vi "Anritsu VNA Set Frequency On-Off.vi"(7 "Anritsu VNA":T1, 8 "error in (no error)":errorcluster, 10 "Blank Frequencies (F)":bool, 11 "VISA Resource Name":refnum<visa-resource-name>) -> (0 "error out":errorcluster, 3 "dup VISA Resource Name":refnum<visa-resource-name>)   [LabVIEW 2011]
doc: "This VI for the HP8753B Network Analyzers reads the stimulus values. Except when performing log sweeps and freq list sweeps, this VI uses the start and stop values and the number of points to calcuate the stimulus values."
uses:
  TypeDefs/Anritsu VNA Instrument Info.ctl
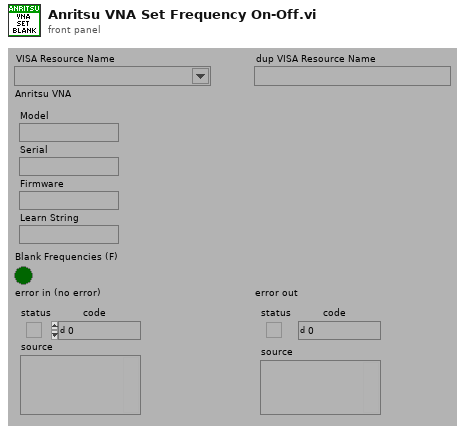
[diagram p1: front panel]
types:
  T1 = typedef "Anritsu VNA Instrument Info.ctl" = cluster{"Model":string, "Serial":string, "Firmware":string, "Learn String":string}
  T2 = typedef "Anritsu VNA Model.ctl" = enum16{"Not Supported", "37XXXX", "MS20XXX", "MS462XX", "MS464XX"}
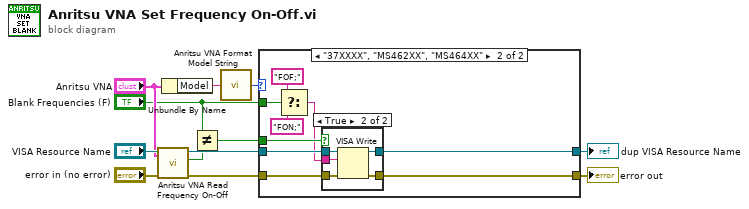
[diagram p0: block diagram]
diagram:
  n1 = call "Anritsu VNA Read Frequency On-Off.vi"("Anritsu VNA"="Anritsu VNA", "error in (no error)"="error in (no error)", "VISA Resource Name"="VISA Resource Name") -> ("error out"=w8:errorcluster, "Frequencies Blanked"=w5:bool, "dup VISA Resource Name"=w9:refnum<visa-resource-name>)  [unwired: 6 out]
  n2 = Unbundle By Name("Anritsu VNA") -> ("Model"=w2:string)
  n3 = Not Equal?(x="Blank Frequencies (F)", y=w5) -> (x != y?=w4:bool)
  n4 = call "Anritsu VNA Format Model String.vi"("Model"=w2) -> ("Model"=w1:T2)
  n5 = case shown="\"37XXXX\", \"MS462XX\", \"MS464XX\"" w1 {
    tunnel: w9 -> [w14 w23]
    tunnel: w8 -> [w13 w22]
    tunnel: [w13 w21] -> w7
    tunnel: [w14 w20] -> w6
    tunnel: w4 -> [_ w19]
    tunnel: "Blank Frequencies (F)" -> [_ w16]
    frame "Not Supported", "MS20XXX" {
      # "These VNAs do not have the ability to blank the frequencies."
    }
    frame "37XXXX", "MS462XX", "MS464XX" {
      n6 = Select(t="FOF;", s=w16, f="FON;") -> (s? t:f=w15:string)
      n7 = case shown="True" w19 {
        tunnel: w23 -> [w25 w30]
        tunnel: w22 -> [w24 w29]
        tunnel: [w24 w28] -> w21
        tunnel: [w25 w27] -> w20
        tunnel: w15 -> [_ w26]
        frame False {
        }
        frame True {
          n8 = VISA Write(VISA resource name=w30, write buffer=w26, error in (no error)=w29) -> (VISA resource name out=w27:refnum<visa-resource-name>, error out=w28:errorcluster)  [unwired: 1 out]
        }
      }
    }
  }
  "dup VISA Resource Name" <- w6
  "error out" <- w7
